vi "getGeneralLocation.vi"(8 "error in (no error)":errorcluster, 11 "Drive in":refnum<class "DriveTo.lvclass">) -> (0 "error out":errorcluster, 2 "General Location":T1 {"North" format="%#_10f"; "East" format="%#_8f"}, 3 "Drive out":refnum<class "DriveTo.lvclass">)   [LabVIEW 2011, in "DriveTo.lvclass"]
uses:
  DriveTo.lvclass
  2 Typedefs/UTM Location.ctl
  DriveTo.lvclass/DriveTo.ctl
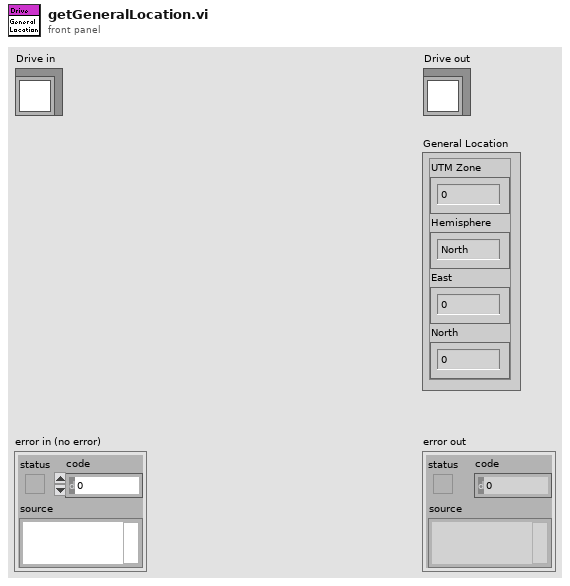
[diagram p1: front panel]
types:
  T1 = typedef "UTM Location.ctl" = cluster{"UTM Zone":dbl, "Hemisphere":enum16{"North", "South"}, "East":dbl, "North":dbl}
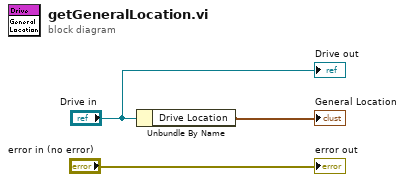
[diagram p0: block diagram]
diagram:
  n1 = Unbundle By Name("Drive in") -> ("Drive Location"=→"General Location":T1)
  "error out" <- "error in (no error)"
  "Drive out" <- "Drive in"
